vi "Build Set.vi"(11 "Example":string) -> (3 "Set":set{i32}(c389))   [LabVIEW 2020]
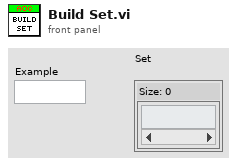
[diagram p1: front panel]
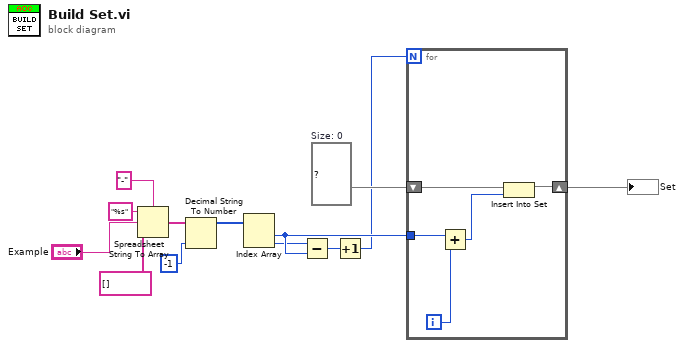
[diagram p0: block diagram]
diagram:
  w10 = set{i32} {}  # Size: 0
  n1 = Spreadsheet String To Array(delimiter (Tab)="-", format string="%s", spreadsheet string="Example", array type (2D Dbl)=string[] [] ("Array")) -> (array=w3:string[])
  n2 = Decimal String To Number(string=w3, default (0L)=-1 ("default (0 I32)")) -> (number=w4:i32[])  [unwired: 1 in, 1 out]
  n3 = Index Array(array=w4) -> (element #1=w9:i32, element #2=w6:i32)  [unwired: 2 in]
  n4 = Subtract(x=w6, y=w9) -> (x-y=w7:i32)
  n5 = Increment(x=w7) -> (x+1=w8:i32)
  n6 = for {
    N: w8 -> [_]
    tunnel: w9 -> [w18]
    shift-right: [w15] -> w11
    shift-left: w10 -> [w14]
    i -> [w17]
    n7 = Add(x=w18, y=w17) -> (x+y=w16:i32)
    n8 = Insert Into Set(10:w16, 11:w14) -> (3:w15:set{i32})  [unwired: 1 out]
  }
  "Set" <- w11
